vi "Old - Move Straight (2).vi"(6 "Angle Reduction Factor":dbl, 8 "error in (no error)":errorcluster, 9 "Encoder Reduction Factor":dbl, 10 "Ref-Nums":T1, 11 "Encoder Distance":dbl=-3600.0 format="%#_13g") -> (0 "error out":errorcluster)   [LabVIEW 2016]
uses:
  <vilib>/Rock Robotics/WPI/Utilities/WPI_GetSetVariantRefNum.vi
panel:
  in  "Reduction Factor 3":dbl
  in  "Encoder Distance 3":dbl=-3600.0 format="%#_13g"
  in  "Reduction Factor 2":dbl
  in  "Encoder Distance 2":dbl=-3600.0 format="%#_13g"
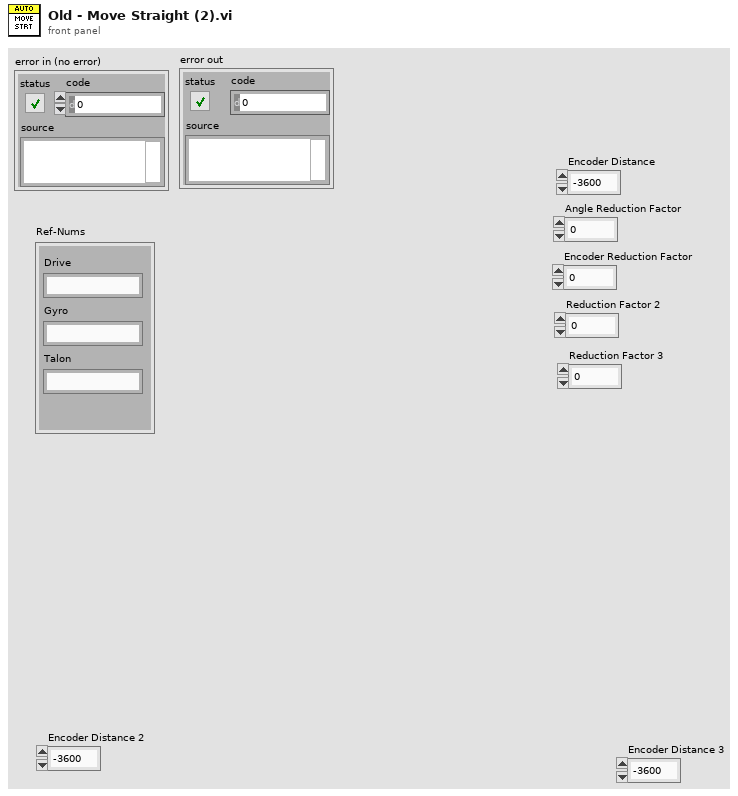
[diagram p1: front panel]
types:
  T1 = cluster{"Drive":string, "Gyro":string, "Talon":string}
  T2 = typedef "WPI_MotorControlDeviceRef.ctl" = cluster{"DeviceStatus":errorcluster, "Type":T3, "PWM":cluster{"PWM Channel":T4, "DeadBand":T5}, "CAN":cluster{"Device Number":u8, "SetOutput VI Ref":variant, "GetOutput VI Ref":variant, "Enable VI Ref":variant, "Disable VI Ref":variant, "Data":variant}, "Invert":bool}
  T3 = typedef "WPI_MotorControlType.ctl" = enum16{"PWM", "CAN"}
  T4 = typedef "FPGA_DIOPWMChannel.ctl" = enum8{"PWM 0", "PWM 1", "PWM 2", "PWM 3", "PWM 4", "PWM 5", "PWM 6", "PWM 7", "PWM 8", "PWM 9", "PWM MXP 0", "PWM MXP 1", "PWM MXP 2", "PWM MXP 3", "PWM MXP 4", "PWM MXP 5", "PWM MXP 6", "PWM MXP 7", "PWM MXP 8", "PWM MXP 9", "Invalid"}
  T5 = typedef "WPI_PWMDeadband.ctl" = cluster{"Name":string, "maxPositivePwm":i32, "minPositivePwm":i32, "centerPwm":i32, "maxNegativePwm":i32, "minNegativePwm":i32, "angularRange":u16}
  T6 = typedef "WPI_CANTalonSRX_GlobalStatus.ctl" = cluster{"Applied Throttle":dbl, "Module Enabled":bool, "CAN Error":errorcluster, "Closed Loop Error":dbl, "Forward Limit Switch Closed":bool, "Reverse Limit Switch Closed":bool, "Sensor Position":dbl, "Sensor Velocity":dbl, "Current":dbl, "Sticky Fault - Over Temp":bool, "Sticky Fault - Under Voltage":bool, "Sticky Fault - Forward Limit":bool, "Sticky Fault - Reverse Limit":bool, "Sticky Fault - Forward Soft Limit":bool, "Sticky Fault - Reverse Soft Limit":bool, "Brake is Enabled":bool, "Encoder Position":dbl, "Encoder Velocity":dbl, "Encoder Index Count":dbl, "Encoder A Pin State":bool, "Encoder B Pin State":bool, "Encoder Index Pin State":bool, "Analog In":dbl, "Analog In Velocity":dbl, "Temperature (C)":dbl, "Battery Voltage":dbl, "Control 5 Is Supported":bool, "Current Profile Slot Select":dbl, "Pos Div 8":bool, "Vel Div 4":bool, "Pulse Width Position":i32, "Pulse Width Velocity":i32, "Pulse Width Rise To Rise (us)":i32, "Pulse Width Rise To Fall (us)":i32, "Mot Prof Active Is Under Run":bool, "Mot Prof Active Has Under Run":bool, "Mot Prof Active Is Last":bool, "Mot Prof Active Velocity Only":bool, "Mot Prof Active Is Valid":bool, "Mot Prof Buffer Is Full":bool, "Mot Prof Active Profile Slot Select":i32, "Mot Prof NextID":i32, "Mot Prof Count":i32, "Mot Prof Active Velocity":dbl, "Mot Prof Active Position":dbl, "Mot Prof Output Enable":i32}
  T7 = typedef "WPI_GyroDevRef.ctl" = cluster{"DevStatus":errorcluster, "Analog Channel":T8, "Offset":dbl, "Gain (VoltsPerDegree/Second)":dbl, "Gyro Type":enum16{"Analog", "XRS450"}, "Handle":i32, "SPI Bus":T9, "Device Found":bool, "Sample Rate":dbl, "Calibrate On Open":bool}
  T8 = typedef "FPGA_AIChannel.ctl" = enum8{"AI 0", "AI 1", "AI 2", "AI 3", "AI MXP 0", "AI MXP 1", "AI MXP 2", "AI MXP 3", "Invalid"}
  T9 = typedef "spi_bus.ctl" = enum16{"SPI On-Board, CS0", "SPI On-Board, CS1", "SPI On-Board, CS2", "SPI On-Board, CS3", "SPI MXP", "Invalid"}
  T10 = typedef "WPI_RobotDriveDevRef.ctl" = cluster{"DevStatus":errorcluster, "Motors[]":T2[], "Square Inputs":bool, "Max Output":dbl}
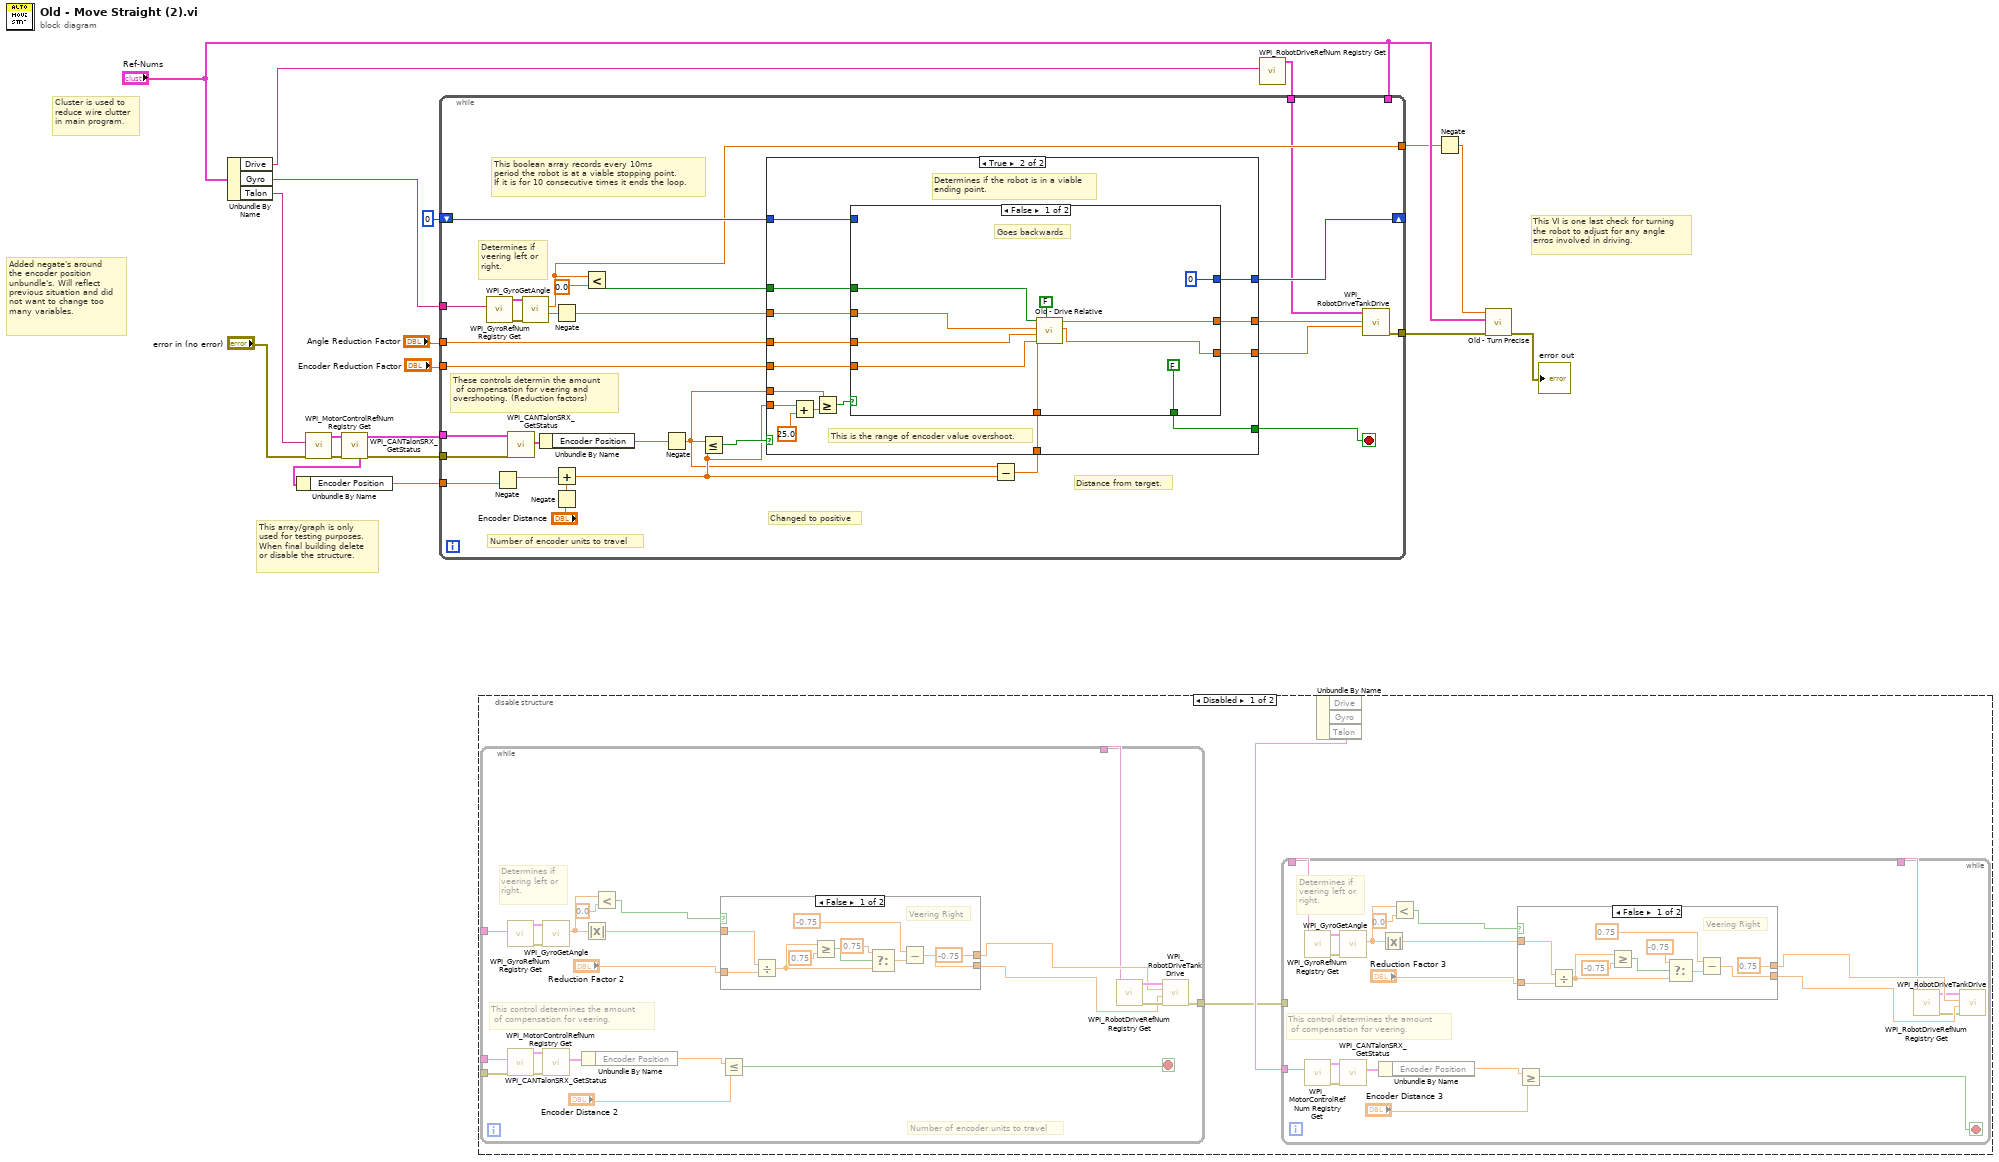
[diagram p0: block diagram]
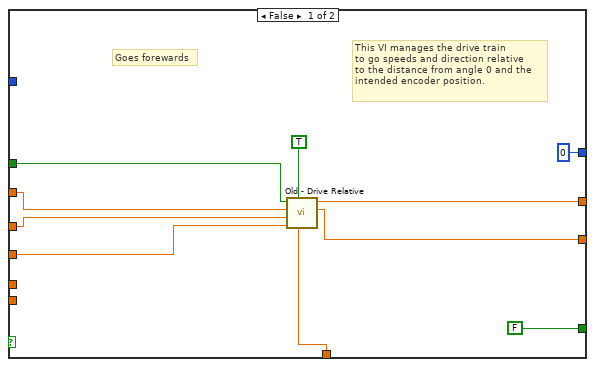
[diagram p2: hidden frame]
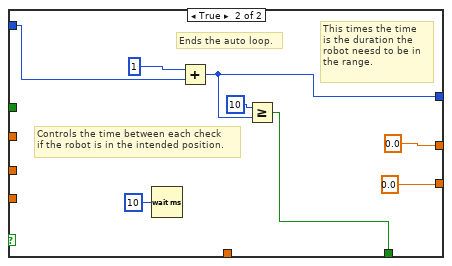
[diagram p3: hidden frame]
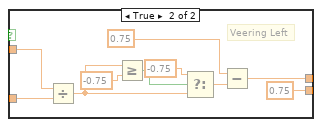
[diagram p4: hidden frame]
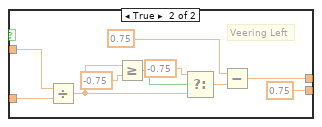
[diagram p5: hidden frame]
diagram:
  # "Added negate's around\nthe encoder position \nunbundle's. Will reflect\nprevious situation and did\nnot want to change too \nmany variables."
  # "This VI is one last check for turning\nthe robot to adjust for any angle \nerros involved in driving."
  # "This array/graph is only\nused for testing purposes.\nWhen final building delete\nor disable the structure."
  # "Cluster is used to\nreduce wire clutter\nin main program."
  n1 = Unbundle By Name("Ref-Nums") -> ("Drive"=w5:string, "Gyro"=w19:string, "Talon"=w10:string)
  n2 = call <vilib>:"WPI_MotorControlRefNum Registry Get.vi"("error in (no error)"="error in (no error)", "refnum name"=w10) -> ("error out"=w12:errorcluster, "MotorControlDevRef"=w11:T2)  [unwired: 8 in]
  n3 = call <vilib>:"WPI_CANTalonSRX_GetStatus.vi"("error in (no error)"=w12, "CAN Talon SRX Ref"=w11) -> ("error out"=w7:errorcluster, "Talon SRX Status"=w3:T6, "CAN Talon SRX Ref"=w8:T2)  [unwired: 7 in]
  n4 = Unbundle By Name(w3) -> ("Encoder Position"=w6:dbl)
  n5 = disable-structure shown="Disabled" {
    frame Disabled {
      n6 = while {
        tunnel: _ -> [w75]
        tunnel: _ -> [w74]
        tunnel: [w73] -> w20
        tunnel: [w72] -> w22
        tunnel: [w67] -> w21
        stop <- w66 stop-if-true
        # "Determines if \nveering left or \nright."
        # "This control determines the amount\n of compensation for veering."
        # "Number of encoder units to travel"
        n7 = call <vilib>:"WPI_GyroRefNum Registry Get.vi"("refnum name"=w74) -> ("error out"=w82:errorcluster, "GyroDevRef"=w83:T7)  [unwired: 9 in]
        n8 = call <vilib>:"WPI_MotorControlRefNum Registry Get.vi"("error in (no error)"=w75, "refnum name"=w73) -> ("error out"=w76:errorcluster, "MotorControlDevRef"=w77:T2)  [unwired: 8 in]
        n9 = call <vilib>:"WPI_GyroGetAngle.vi"("error in"=w82, "GyroDevRef"=w83) -> ("Angle"=w81:dbl)  [unwired: 5 in, 4 out]
        n10 = call <vilib>:"WPI_CANTalonSRX_GetStatus.vi"("error in (no error)"=w76, "CAN Talon SRX Ref"=w77) -> ("Talon SRX Status"=w78:T6)  [unwired: 7 in, 2 out]
        n11 = Unbundle By Name(w78) -> ("Encoder Position"=w71:dbl)
        n12 = Absolute Value(x=w81) -> (abs(x)=w85:dbl)
        n13 = Less?(x=w81, y=0.0) -> (x < y?=w86:bool)
        n14 = case shown="False" w86 {
          tunnel: [-0.75 w101] -> w69
          tunnel: [w90 0.75] -> w68
          tunnel: w85 -> [w89 w99]
          tunnel: "Reduction Factor 2" -> [w88 w98]
          frame False {
            # "Veering Right"
            n15 = Divide(x=w89, y=w88) -> (x/y=w92:dbl)
            n16 = Greater Or Equal?(x=w92, y=0.75) -> (x >= y?=w96:bool)
            n17 = Select(t=0.75, s=w96, f=w92) -> (s? t:f=w93:dbl)
            n18 = Subtract(x=-0.75 ("y"), y=w93) -> (x-y=w90:dbl)
          }
          frame True {
            # "Veering Left"
            n19 = Divide(x=w99, y=w98) -> (x/y=w102:dbl)
            n20 = Greater Or Equal?(x=w102, y=-0.75) -> (x >= y?=w106:bool)
            n21 = Select(t=-0.75, s=w106, f=w102) -> (s? t:f=w103:dbl)
            n22 = Subtract(x=0.75 ("y"), y=w103) -> (x-y=w101:dbl)
          }
        }
        n23 = Less Or Equal?(x=w71, y="Encoder Distance 2") -> (x <= y?=w66:bool)
        n24 = call <vilib>:"WPI_RobotDriveRefNum Registry Get.vi"("refnum name"=w67) -> ("error out"=w80:errorcluster, "RobotDriveDevRef"=w79:T10)  [unwired: 9 in]
        n25 = call <vilib>:"WPI_RobotDriveTankDrive.vi"("error in (no error)"=w80, "Right axis value"=w68, "Left axis value"=w69, "RobotDriveDevRef"=w79) -> ("error out"=w72:errorcluster)  [unwired: 5 in, 2 out]
      }
      n26 = Unbundle By Name() -> ("Talon"=w25:string)  [unwired: 1 in, 2 out]
      n27 = while {
        tunnel: w22 -> [_]
        tunnel: [w28] -> w23
        tunnel: [w27] -> w24
        tunnel: w25 -> [w26]
        stop <- w29 stop-if-true
        # "Determines if \nveering left or \nright."
        # "This control determines the amount\n of compensation for veering."
        n28 = call <vilib>:"WPI_GyroRefNum Registry Get.vi"("refnum name"=w27) -> ("error out"=w35:errorcluster, "GyroDevRef"=w34:T7)  [unwired: 9 in]
        n29 = call <vilib>:"WPI_MotorControlRefNum Registry Get.vi"("refnum name"=w26) -> ("error out"=w41:errorcluster, "MotorControlDevRef"=w40:T2)  [unwired: 9 in]
        n30 = call <vilib>:"WPI_GyroGetAngle.vi"("error in"=w35, "GyroDevRef"=w34) -> ("Angle"=w36:dbl)  [unwired: 5 in, 4 out]
        n31 = call <vilib>:"WPI_CANTalonSRX_GetStatus.vi"("error in (no error)"=w41, "CAN Talon SRX Ref"=w40) -> ("Talon SRX Status"=w39:T6)  [unwired: 7 in, 2 out]
        n32 = Unbundle By Name(w39) -> ("Encoder Position"=w42:dbl)
        n33 = Absolute Value(x=w36) -> (abs(x)=w32:dbl)
        n34 = Less?(x=w36, y=0.0) -> (x < y?=w31:bool)
        n35 = case shown="False" w31 {
          tunnel: [0.75 w59] -> w44
          tunnel: [w48 0.75] -> w45
          tunnel: w32 -> [w47 w57]
          tunnel: "Reduction Factor 3" -> [w46 w56]
          frame False {
            # "Veering Right"
            n36 = Divide(x=w47, y=w46) -> (x/y=w50:dbl)
            n37 = Greater Or Equal?(x=w50, y=-0.75) -> (x >= y?=w54:bool)
            n38 = Select(t=-0.75, s=w54, f=w50) -> (s? t:f=w51:dbl)
            n39 = Subtract(x=0.75 ("y"), y=w51) -> (x-y=w48:dbl)
          }
          frame True {
            # "Veering Left"
            n40 = Divide(x=w57, y=w56) -> (x/y=w60:dbl)
            n41 = Greater Or Equal?(x=w60, y=-0.75) -> (x >= y?=w64:bool)
            n42 = Select(t=-0.75, s=w64, f=w60) -> (s? t:f=w61:dbl)
            n43 = Subtract(x=0.75 ("y"), y=w61) -> (x-y=w59:dbl)
          }
        }
        n44 = Greater Or Equal?(x=w42, y="Encoder Distance 3") -> (x >= y?=w29:bool)
        n45 = call <vilib>:"WPI_RobotDriveRefNum Registry Get.vi"("refnum name"=w28) -> ("error out"=w37:errorcluster, "RobotDriveDevRef"=w38:T10)  [unwired: 9 in]
        n46 = call <vilib>:"WPI_RobotDriveTankDrive.vi"("error in (no error)"=w37, "Right axis value"=w45, "Left axis value"=w44, "RobotDriveDevRef"=w38) -> ()  [unwired: 5 in, 3 out]
      }
    }
    frame Enabled {
    }
  }
  n47 = call <vilib>:"WPI_RobotDriveRefNum Registry Get.vi"("refnum name"=w5) -> ("RobotDriveDevRef"=w4:T10)  [unwired: 9 in, 1 out]
  n48 = while {
    tunnel: w19 -> [w132]
    tunnel: w8 -> [w122]
    tunnel: [w131] -> w14
    tunnel: w7 -> [w121]
    shift-right: [w126] -> _
    shift-left: 0 -> [w125]
    tunnel: [w123] -> w16
    tunnel: "Ref-Nums" -> [_]
    tunnel: w6 -> [w108]
    tunnel: w4 -> [w118]
    tunnel: "Angle Reduction Factor" -> [w117]
    tunnel: "Encoder Reduction Factor" -> [w116]
    stop <- w129 stop-if-true
    # "Changed to positive"
    # "Distance from target."
    # "This boolean array records every 10ms\nperiod the robot is at a viable stopping point.\nIf it is for 10 consecutive times it ends the loop."
    # "Determines if \nveering left or \nright."
    # "These controls determin the amount\n of compensation for veering and \novershooting. (Reduction factors)"
    # "Number of encoder units to travel"
    n49 = call <vilib>:"WPI_GyroRefNum Registry Get.vi"("refnum name"=w132) -> ("error out"=w133:errorcluster, "GyroDevRef"=w134:T7)  [unwired: 9 in]
    n50 = Negate(x=w108) -> (-x=w109:dbl)
    n51 = call <vilib>:"WPI_CANTalonSRX_GetStatus.vi"("error in (no error)"=w121, "CAN Talon SRX Ref"=w122) -> ("Talon SRX Status"=w120:T6)  [unwired: 7 in, 2 out]
    n52 = call <vilib>:"WPI_GyroGetAngle.vi"("error in"=w133, "GyroDevRef"=w134) -> ("Angular Rate"=w114:dbl, "Angle"=w123:dbl)  [unwired: 5 in, 3 out]
    n53 = Unbundle By Name(w120) -> ("Encoder Position"=w112:dbl)
    n54 = Negate(x=w114) -> (-x=w115:dbl)
    n55 = Negate(x="Encoder Distance") -> (-x=w111:dbl)
    n56 = Add(x=w109, y=w111) -> (x+y=w119:dbl)
    n57 = Less?(x=w123, y=0.0) -> (x < y?=w135:bool)
    n58 = Negate(x=w112) -> (-x=w113:dbl)
    n59 = Less Or Equal?(x=w113, y=w119) -> (x <= y?=w130:bool)
    n60 = Subtract(x=w113, y=w119) -> (x-y=w124:dbl)
    n61 = case shown="True" w130 {
      tunnel: w135 -> [w146 w161]
      tunnel: w115 -> [w145 w160]
      tunnel: w117 -> [w144 w159]
      tunnel: w113 -> [_ w157]
      tunnel: [w143 w153] -> w128
      tunnel: [w142 w152] -> w127
      tunnel: [FALSE w154] -> w129
      tunnel: [0 w151] -> w126
      tunnel: w125 -> [_ w150]
      tunnel: w119 -> [_ w149]
      tunnel: w124 -> [w139 w147]
      tunnel: w116 -> [w138 w148]
      frame False {
        # "This VI manages the drive train\nto go speeds and direction relative\nto the distance from angle 0 and the\nintended encoder position."
        # "Goes forewards"
        n62 = call "Old - Drive Relative.vi"("Distance From Target"=w139, "Encoder Direction"=TRUE, "Encoder Reduction Factor"=w138, "Angle Reduction Factor"=w144, "Angle"=w145, "Angle Direction"=w146) -> ("Right Power"=w142:dbl, "Left Power"=w143:dbl)  [unwired: 4 in]
      }
      frame True {
        # "This is the range of encoder value overshoot."
        # "Determines if the robot is in a viable\nending point."
        n63 = Add(x=w149, y=25.0) -> (x+y=w155:dbl)
        n64 = Greater Or Equal?(x=w157, y=w155) -> (x >= y?=w158:bool)
        n65 = case shown="False" w158 {
          tunnel: w161 -> [w169 _]
          tunnel: w160 -> [w168 _]
          tunnel: w159 -> [w167 _]
          tunnel: [FALSE w172] -> w154
          tunnel: [w163 0.0] -> w153
          tunnel: [w164 0.0] -> w152
          tunnel: [0 w174] -> w151
          tunnel: w150 -> [_ w175]
          tunnel: w148 -> [w166 _]
          tunnel: w147 -> [w165 _]
          frame False {
            # "Goes backwards"
            n66 = call "Old - Drive Relative.vi"("Distance From Target"=w165, "Encoder Direction"=FALSE, "Encoder Reduction Factor"=w166, "Angle Reduction Factor"=w167, "Angle"=w168, "Angle Direction"=w169) -> ("Right Power"=w164:dbl, "Left Power"=w163:dbl)  [unwired: 4 in]
          }
          frame True {
            # "This times the time\nis the duration the \nrobot neesd to be in \nthe range."
            # "Controls the time between each check\nif the robot is in the intended position."
            # "Ends the auto loop."
            n67 = Wait (ms)(milliseconds to wait=u32 10) -> ()  [unwired: 1 out]
            n68 = Add(x=1, y=w175) -> (x+y=w174:i32)
            n69 = Greater Or Equal?(x=10, y=w174) -> (x >= y?=w172:bool)
          }
        }
      }
    }
    n70 = call <vilib>:"WPI_RobotDriveTankDrive.vi"("Right axis value"=w127, "Left axis value"=w128, "RobotDriveDevRef"=w118) -> ("error out"=w131:errorcluster)  [unwired: 6 in, 2 out]
  }
  n71 = Negate(x=w16) -> (-x=w15:dbl)
  n72 = call "Old - Turn Precise.vi"("error in (no error)"=w14, "Ref-Nums"="Ref-Nums", "Angle"=w15) -> ("error out"=→"error out":errorcluster)  [unwired: 8 in]
